vi "CameraStartAcquire.vi"(8 "error in (no error)":errorcluster, 11 "AndorSDK2 in":refnum<class "Andor2.lvclass">) -> (0 "error out":errorcluster, 3 "AndorSDK2 out":refnum<class "Andor2.lvclass">)   [LabVIEW 2010, in "Andor2.lvclass"]
uses:
  Andor2.lvclass
  <userlib>/Andor/atmcd32d.llb/Shutter_type typedef.ctl
  <userlib>/Andor/atmcd32d.llb/Shutter_mode typedef.ctl
  Andor2.lvclass/Andor2.ctl
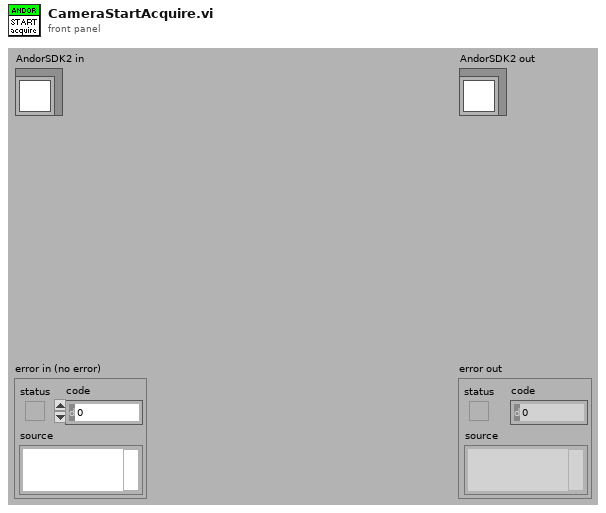
[diagram p1: front panel]
types:
  T1 = typedef "Shutter_mode typedef.ctl" = enum16{"Auto", "Open", "Close"}
  T2 = typedef "Shutter_type typedef.ctl" = enum16{"TTL Low", "TTL High"}
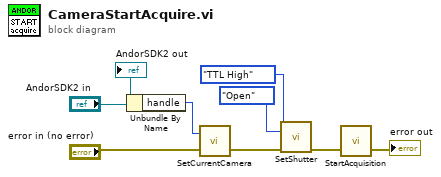
[diagram p0: block diagram]
diagram:
  n1 = Unbundle By Name("AndorSDK2 in") -> ("handle"=w7:i32)
  n2 = call <userlib>:"SetCurrentCamera.vi"("error in (no error)"="error in (no error)", "cameraHandle"=w7) -> ("error out"=w5:errorcluster)  [unwired: 1 out]
  n3 = call <userlib>:"SetShutter.vi"("type"=Shutter_type_typedef."TTL High", "mode"=Shutter_mode_typedef."Open", "error in (no error)"=w5) -> ("error out"=w2:errorcluster)  [unwired: 11 in, 1 out]
  n4 = call <userlib>:"StartAcquisition.vi"("error in (no error)"=w2) -> ("error out"=→"error out":errorcluster)  [unwired: 1 in, 1 out]
  "AndorSDK2 out" <- "AndorSDK2 in"
